vi "Post Build Script.vi"(8 "error in (no error)":errorcluster, 11 "PostBuildSupport in":refnum<class "PostBuildSupport.lvclass">) -> (0 "error out":errorcluster)   [LabVIEW 2016, in "PostBuildSupport.lvclass"]
uses:
  PostBuildSupport.lvclass
  <vilib>/addons/WireFlow/_WF_ProgressBar.llb/ProgressBar_WireFlow.lvclass
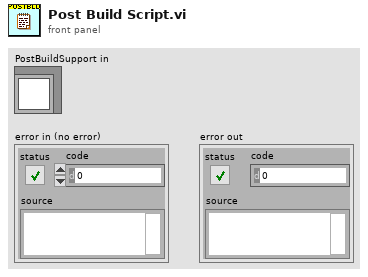
[diagram p1: front panel]
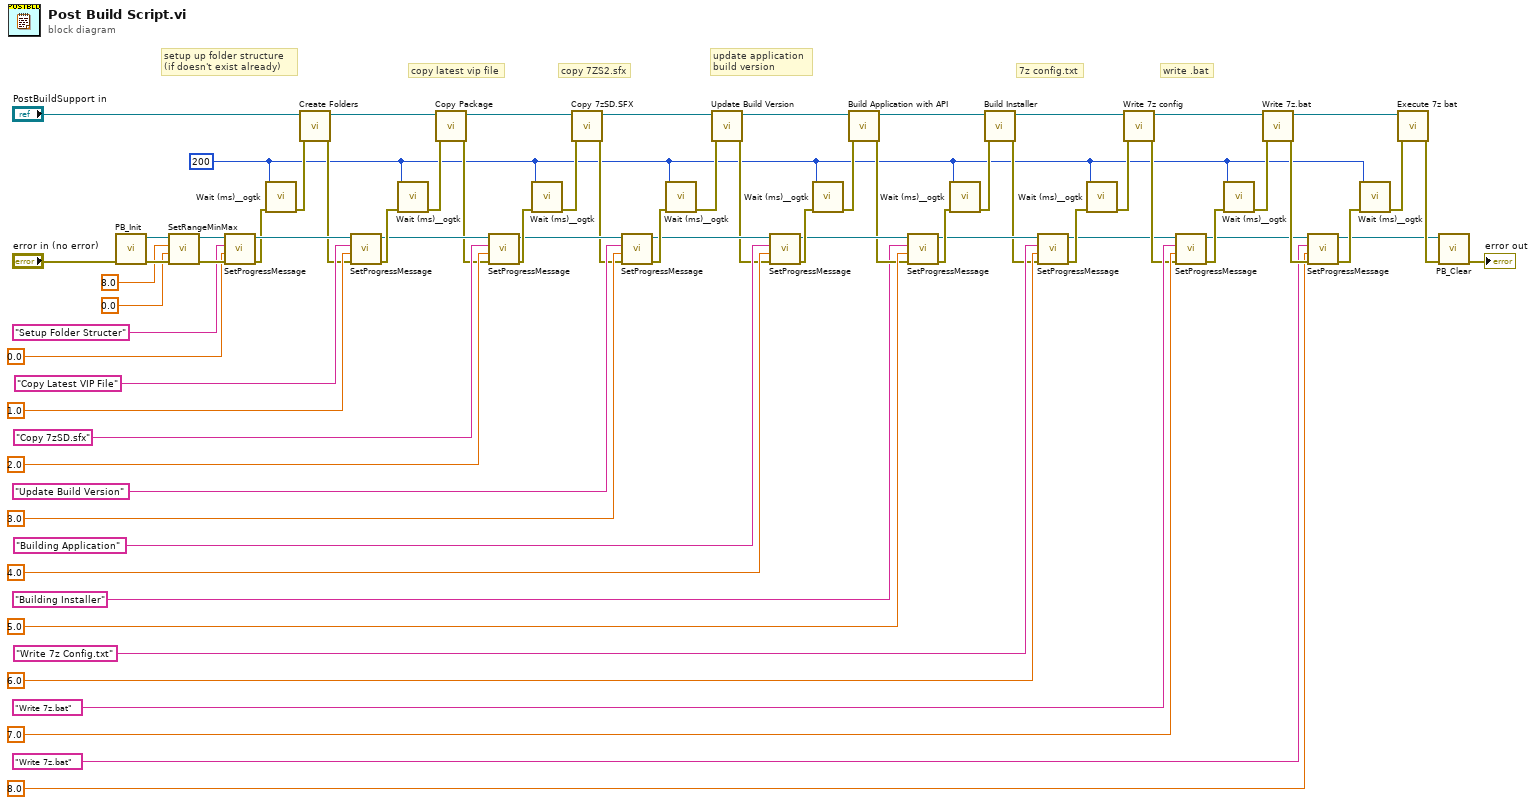
[diagram p0: block diagram]
diagram:
  w1 = u32 200 ("milliseconds to wait")
  # "copy 7ZS2.sfx"
  # "setup up folder structure \n(if doesn't exist already)"
  # "update application\nbuild version"
  # "copy latest vip file"
  # "7z config.txt"
  # "write .bat"
  n1 = call <vilib>:"PB_Init.vi"("error in (no error)"="error in (no error)") -> ("error out"=w63:errorcluster, "WF-ProgressBar out"=w31:refnum<class "ProgressBar_WireFlow.lvclass">)  [unwired: 9 in]
  n2 = call-dynamic "SetRangeMinMax.vi"("error in (no error)"=w63, "Min (0)"=0.0, "Max (1)"=8.0, "WF-ProgressBar in"=w31) -> ("error out"=w61:errorcluster, "WF-ProgressBar out"=w32:refnum<class "ProgressBar_WireFlow.lvclass">)  [unwired: 6 in]
  n3 = call-dynamic "SetProgressMessage.vi"("error in (no error)"=w61, "Progress value (NaN no update)"=0.0, "Message"="Setup Folder Structer", "WF-ProgressBar in"=w32) -> ("error out"=w27:errorcluster, "WF-ProgressBar out"=w39:refnum<class "ProgressBar_WireFlow.lvclass">)  [unwired: 5 in, 1 out]
  n4 = call <userlib>:"Wait (ms)__ogtk.vi"("error in (no error)"=w27, "milliseconds to wait"=w1) -> ("error out"=w10:errorcluster)  [unwired: 8 in, 1 out]
  n5 = call "Create Folders.vi"("error in (no error)"=w10, "PostBuildSupport in"="PostBuildSupport in") -> ("error out"=w26:errorcluster, "PostBuildSupport out"=w70:refnum<class "PostBuildSupport.lvclass">)  [unwired: 8 in]
  n6 = call-dynamic "SetProgressMessage.vi"("error in (no error)"=w26, "Progress value (NaN no update)"=1.0, "Message"="Copy Latest VIP File", "WF-ProgressBar in"=w39) -> ("error out"=w58:errorcluster, "WF-ProgressBar out"=w30:refnum<class "ProgressBar_WireFlow.lvclass">)  [unwired: 5 in, 1 out]
  n7 = call <userlib>:"Wait (ms)__ogtk.vi"("error in (no error)"=w58, "milliseconds to wait"=w1) -> ("error out"=w9:errorcluster)  [unwired: 8 in, 1 out]
  n8 = call "Copy Package.vi"("error in (no error)"=w9, "PostBuildSupport in"=w70) -> ("error out"=w29:errorcluster, "PostBuildSupport out"=w69:refnum<class "PostBuildSupport.lvclass">)  [unwired: 8 in]
  n9 = call-dynamic "SetProgressMessage.vi"("error in (no error)"=w29, "Progress value (NaN no update)"=2.0, "Message"="Copy 7zSD.sfx", "WF-ProgressBar in"=w30) -> ("error out"=w45:errorcluster, "WF-ProgressBar out"=w38:refnum<class "ProgressBar_WireFlow.lvclass">)  [unwired: 5 in, 1 out]
  n10 = call <userlib>:"Wait (ms)__ogtk.vi"("error in (no error)"=w45, "milliseconds to wait"=w1) -> ("error out"=w8:errorcluster)  [unwired: 8 in, 1 out]
  n11 = call "Copy 7zSD.SFX.vi"("error in (no error)"=w8, "PostBuildSupport in"=w69) -> ("error out"=w28:errorcluster, "PostBuildSupport out"=w68:refnum<class "PostBuildSupport.lvclass">)  [unwired: 8 in]
  n12 = call-dynamic "SetProgressMessage.vi"("error in (no error)"=w28, "Progress value (NaN no update)"=3.0, "Message"="Update Build Version", "WF-ProgressBar in"=w38) -> ("error out"=w44:errorcluster, "WF-ProgressBar out"=w37:refnum<class "ProgressBar_WireFlow.lvclass">)  [unwired: 5 in, 1 out]
  n13 = call <userlib>:"Wait (ms)__ogtk.vi"("error in (no error)"=w44, "milliseconds to wait"=w1) -> ("error out"=w7:errorcluster)  [unwired: 8 in, 1 out]
  n14 = call "Update Build Version.vi"("error in (no error)"=w7, "PostBuildSupport in"=w68) -> ("error out"=w16:errorcluster, "PostBuildSupport out"=w67:refnum<class "PostBuildSupport.lvclass">)  [unwired: 8 in]
  n15 = call-dynamic "SetProgressMessage.vi"("error in (no error)"=w16, "Progress value (NaN no update)"=4.0, "Message"="Building Application", "WF-ProgressBar in"=w37) -> ("error out"=w43:errorcluster, "WF-ProgressBar out"=w36:refnum<class "ProgressBar_WireFlow.lvclass">)  [unwired: 5 in, 1 out]
  n16 = call <userlib>:"Wait (ms)__ogtk.vi"("error in (no error)"=w43, "milliseconds to wait"=w1) -> ("error out"=w6:errorcluster)  [unwired: 8 in, 1 out]
  n17 = call "Build Application with API.vi"("error in (no error)"=w6, "PostBuildSupport in"=w67) -> ("error out"=w15:errorcluster, "PostBuildSupport out"=w65:refnum<class "PostBuildSupport.lvclass">)  [unwired: 8 in]
  n18 = call-dynamic "SetProgressMessage.vi"("error in (no error)"=w15, "Progress value (NaN no update)"=5.0, "Message"="Building Installer", "WF-ProgressBar in"=w36) -> ("error out"=w42:errorcluster, "WF-ProgressBar out"=w35:refnum<class "ProgressBar_WireFlow.lvclass">)  [unwired: 5 in, 1 out]
  n19 = call <userlib>:"Wait (ms)__ogtk.vi"("error in (no error)"=w42, "milliseconds to wait"=w1) -> ("error out"=w5:errorcluster)  [unwired: 8 in, 1 out]
  n20 = call "Build Installer.vi"("error in (no error)"=w5, "PostBuildSupport in"=w65) -> ("error out"=w13:errorcluster, "PostBuildSupport out"=w66:refnum<class "PostBuildSupport.lvclass">)  [unwired: 8 in]
  n21 = call-dynamic "SetProgressMessage.vi"("error in (no error)"=w13, "Progress value (NaN no update)"=6.0, "Message"="Write 7z Config.txt", "WF-ProgressBar in"=w35) -> ("error out"=w41:errorcluster, "WF-ProgressBar out"=w34:refnum<class "ProgressBar_WireFlow.lvclass">)  [unwired: 5 in, 1 out]
  n22 = call <userlib>:"Wait (ms)__ogtk.vi"("error in (no error)"=w41, "milliseconds to wait"=w1) -> ("error out"=w4:errorcluster)  [unwired: 8 in, 1 out]
  n23 = call "Write 7z config.vi"("error in (no error)"=w4, "PostBuildSupport in"=w66) -> ("error out"=w40:errorcluster, "PostBuildSupport out"=w71:refnum<class "PostBuildSupport.lvclass">)  [unwired: 8 in]
  n24 = call-dynamic "SetProgressMessage.vi"("error in (no error)"=w40, "Progress value (NaN no update)"=7.0, "Message"="Write 7z.bat", "WF-ProgressBar in"=w34) -> ("error out"=w33:errorcluster, "WF-ProgressBar out"=w24:refnum<class "ProgressBar_WireFlow.lvclass">)  [unwired: 5 in, 1 out]
  n25 = call <userlib>:"Wait (ms)__ogtk.vi"("error in (no error)"=w33, "milliseconds to wait"=w1) -> ("error out"=w3:errorcluster)  [unwired: 8 in, 1 out]
  n26 = call "Write 7z.bat.vi"("error in (no error)"=w3, "PostBuildSupport in"=w71) -> ("error out"=w25:errorcluster, "PostBuildSupport out"=w22:refnum<class "PostBuildSupport.lvclass">)  [unwired: 8 in]
  n27 = call-dynamic "SetProgressMessage.vi"("error in (no error)"=w25, "Progress value (NaN no update)"=8.0, "Message"="Write 7z.bat", "WF-ProgressBar in"=w24) -> ("error out"=w23:errorcluster, "WF-ProgressBar out"=w18:refnum<class "ProgressBar_WireFlow.lvclass">)  [unwired: 5 in, 1 out]
  n28 = call <userlib>:"Wait (ms)__ogtk.vi"("error in (no error)"=w23, "milliseconds to wait"=w1) -> ("error out"=w2:errorcluster)  [unwired: 8 in, 1 out]
  n29 = call "Execute 7z bat.vi"("error in (no error)"=w2, "PostBuildSupport in"=w22) -> ("error out"=w19:errorcluster)  [unwired: 8 in, 1 out]
  n30 = call-dynamic "PB_Clear.vi"("error in (no error)"=w19, "WF-ProgressBar in"=w18) -> ("error out"=→"error out":errorcluster)  [unwired: 8 in, 1 out]
